vi "PH_OceanOpticsSpectrometer.PC write PSDB.vi"(0 "i ref in":refnum<vi>, 5 "error IO":errorcluster) -> (14 "i ref out":refnum<vi>, 19 "error out":errorcluster)   [LabVIEW 2014, in "PH_OceanOpticsSpectrometer.lvlib"]
doc: "This is the proc case which writes data to the PHELIX shot data base."
uses:
  PH_OceanOpticsSpectrometer.lvlib
  CSlibraries-extern/psdb_lv/PSDB_AxisDescription.ctl
  PH_Basics/PH_PSDBWriter/PH_PSDBWriter.2D dataset.ctl
  PH_Basics/PH_Common/PH_Common.lvlib
  PH_Basics/PH_PSDBWriter/PH_PSDBWriter.lvlib
  CSlibraries-extern/psdb_lv/PSDB.lvlib
  PH_Basics/PH_StatusHandler/PH_StatusHandler.lvlib
panel:
  in  "axis description":T1={"x axis label"="Wavelength", "y axis label"="nm", "x axis unit"="Counts", "y axis unit"="#"}
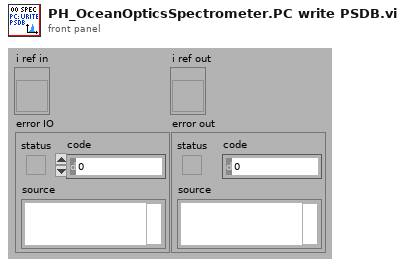
[diagram p1: front panel]
types:
  T1 = typedef "PSDB.lvlib/PSDB_AxisDescription.ctl" = cluster{"x axis label":string, "y axis label":string, "x axis unit":string, "y axis unit":string}
  T2 = typedef "PH_PSDBWriter.lvlib/PH_PSDBWriter.2D dataset.ctl" = cluster{"name":string, "data":dbl[][], "axis description":T1}
  T3 = typedef "PH_OceanOpticsSpectrometer.lvlib/PH_OceanOpticsSpectrometer.i attribute.ctl" = cluster{"GUI Refs":cluster{"Delete":refnum<vi>, "Spectrum":refnum<vi>, "Display Width":refnum<vi>, "Display Center":refnum<vi>, "Save":refnum<vi>, "Integration time":refnum<vi>, "center wavelength":refnum<vi>, "width":refnum<vi>, "Wanted Trigger Mode":refnum<vi>, "Current Trigger Mode":refnum<vi>, "Trigger Info":refnum<vi>, "Model":refnum<vi>, "Driver":refnum<vi>, "Firmware":refnum<vi>}, "Display":cluster{"Width":dbl, "Center":dbl}, "VISA resource name":refnum<visa-resource-name>, "Integration time [ms]":cluster{"Current Value":u16, "Wanted Value":u16}, "Trigger":cluster{"Current value":T4, "Wanted value":T4}, "Default VISA Timeout":u32, "Last Data":cluster{"Wavelength Bins":dbl[], "Spectrum by Pixels":dbl[]}}
  T4 = typedef "PH_OceanOpticsSpectrometer.lvlib/PH_OceanOpticsSpectrometer.Trigger.ctl" = enum32{"External", "Normal"}
  T5 = typedef "PH_PSDBWriter.lvlib/PH_PSDBWriter.Numeric dataset.ctl" = cluster{"name":string, "data":dbl, "unit":string}
  T6 = typedef "PH_PSDBWriter.lvlib/PH_PSDBWriter.String dataset.ctl" = cluster{"name":string, "data":string, "unit":string}
  T7 = typedef "PH_PSDBWriter.lvlib/PH_PSDBWriter.PSDB Dataset.ctl" = cluster{"Version":i32, "2D data Input":T2[], "Boolean Input":T8[], "Image Input":T9[], "Numeric Input":T5[], "String Input":T6[]}
  T8 = typedef "PH_PSDBWriter.lvlib/PH_PSDBWriter.Boolean dataset.ctl" = cluster{"name":string, "data":bool, "unit":string}
  T9 = typedef "PH_PSDBWriter.lvlib/PH_PSDBWriter.Image dataset.ctl" = cluster{"name":string, "data":T10, "unit":string}
  T10 = typedef "IMAQ Image.ctl" = refnum<image>
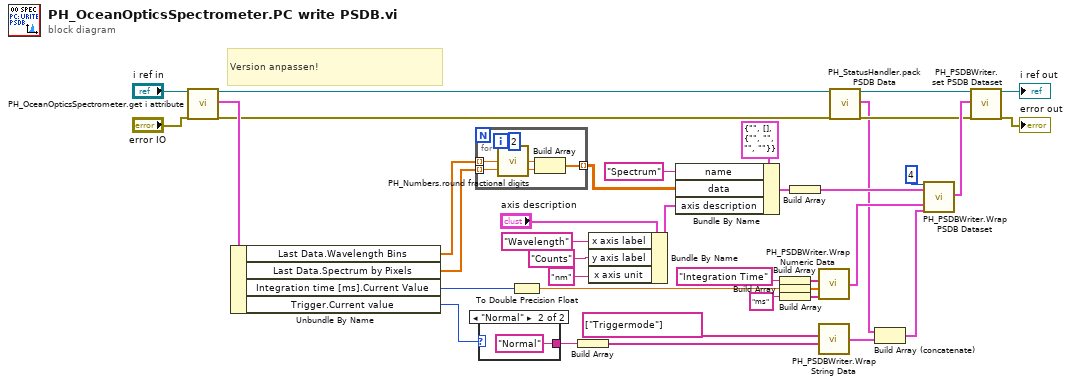
[diagram p0: block diagram]
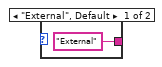
[diagram p2: hidden frame]
diagram:
  # "Version anpassen!"
  n1 = call "PH_OceanOpticsSpectrometer.get i attribute.vi"("i ref in"="i ref in", "error in (no error)"="error IO") -> ("i ref out"=w4:refnum<vi>, "i attribute"=w28:T3, "error out"=w27:errorcluster)  [unwired: 15 in]
  n2 = Unbundle By Name(w28) -> ("Last Data.Wavelength Bins"=w36:dbl[], "Last Data.Spectrum by Pixels"=w35:dbl[], "Integration time [ms].Current Value"=w30:u16, "Trigger.Current value"=w29:T4)
  n3 = for {
    tunnel: w36 -> [w42] mode=indexing
    tunnel: w35 -> [w39] mode=indexing
    tunnel: [w43] -> w23 mode=indexing
    n4 = call "PH_Numbers.round fractional digits.vi"("Input"=w42, "Position (1)"=i16 2) -> ("round Output"=w41:dbl)
    n5 = Build Array(w41, w39) -> (w43:dbl[])
  }
  n6 = case shown="\"Normal\"" w29 {
    tunnel: ["External" ("unit") "Normal" ("unit")] -> w26
    frame "External", Default {
    }
    frame "Normal" {
    }
  }
  n7 = To Double Precision Float(number=w30) -> (double precision float=w12:dbl)
  n8 = Build Array(w26) -> (w8:string[])
  n9 = Bundle By Name(cluster="axis description", "x axis label"="Wavelength", "y axis label"="Counts" ("x axis unit"), "x axis unit"="nm" ("y axis label")) -> (w22:T1)
  n10 = Bundle By Name(cluster=T2 {"name"="", "data"=[], "axis description"={"x axis label"="", "y axis label"="", "x axis unit"="", "y axis unit"=""}} ("2D data"), "name"="Spectrum", "data"=w23, "axis description"=w22) -> (w21:T2)
  n11 = Build Array("Integration Time" ("name")) -> (w9:string[])
  n12 = Build Array(w12) -> (w11:dbl[])
  n13 = Build Array("ms" ("unit")) -> (w10:string[])
  n14 = Build Array(w21) -> (w16:T2[])
  n15 = call "PH_PSDBWriter.Wrap Numeric Data.vi"("Unit Array"=w10, "Data Array"=w11, "Name Array"=w9) -> ("PSDB Numeric Data Array"=w15:T5[])  [unwired: 1 in]
  n16 = call "PH_PSDBWriter.Wrap String Data.vi"("Data Array"=w8, "Name Array"=string[] ["Triggermode"]) -> ("PSDB String Data Array"=w6:T6[])  [unwired: 2 in]
  n17 = call "PH_StatusHandler.pack PSDB Data.vi"("VI in"=w4, "error in (no error)"=w27) -> ("VI out"=w3:refnum<vi>, "PSDB String Data Array"=w1:T6[], "error out"=w5:errorcluster)  [unwired: 15 in]
  n18 = Build Array (concatenate)(w1, w6) -> (w2:T6[])
  n19 = call "PH_PSDBWriter.Wrap PSDB Dataset.vi"("Version"=4, "2D data Input"=w16, "Numeric Input"=w15, "String Input"=w2) -> ("PSDB Dataset"=w18:T7)  [unwired: 15 in]
  n20 = call "PH_PSDBWriter.set PSDB Dataset.vi"("VI in"=w3, "PSDB Dataset"=w18, "error in (no error)"=w5) -> ("VI out"=→"i ref out":refnum<vi>, "error out"=→"error out":errorcluster)  [unwired: 15 in]
